vi "Interpolate.vi"(9 "offset":dbl, 10 "Target dt":dbl, 11 "input waveform":waveform(dbl)) -> (3 "output waveform":waveform(dbl))   [LabVIEW 2018, in "Waveform Equalizer.lvlib"]
uses:
  Waveform Equalizer.lvlib
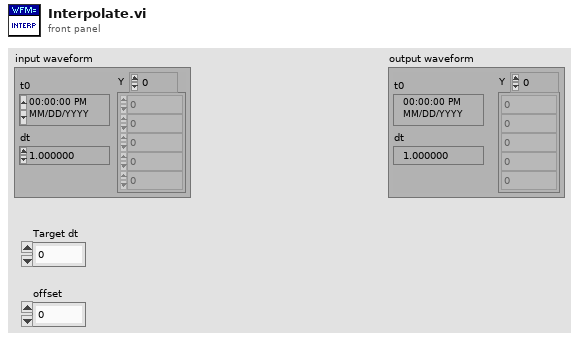
[diagram p1: front panel]
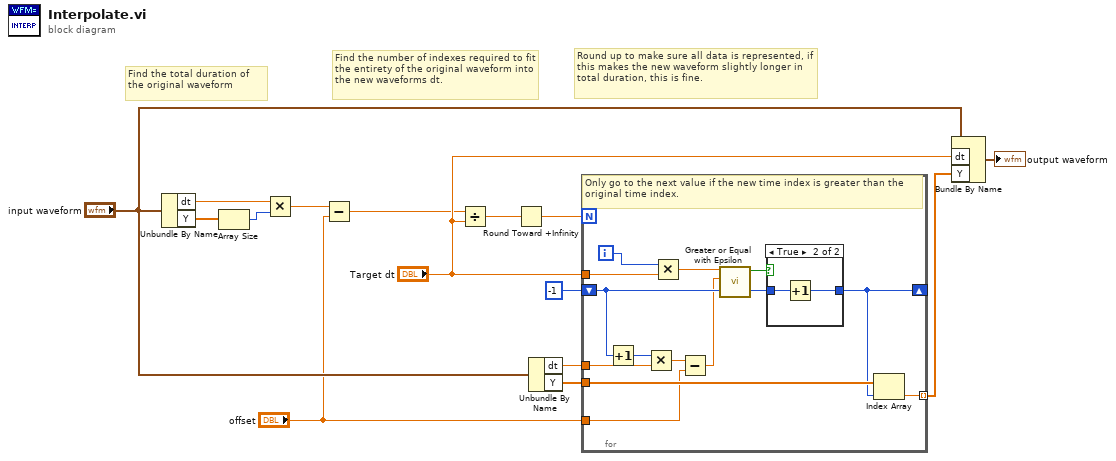
[diagram p0: block diagram]
diagram:
  # "Round up to make sure all data is represented, if this makes the new waveform slightly longer in total duration, this is fine."
  # "Find the number of indexes required to fit the entirety of the original waveform into the new waveforms dt."
  # "Find the total duration of the original waveform"
  n1 = Unbundle By Name("input waveform") -> ("dt"=w13:dbl, "Y"=w15:dbl[])
  n2 = Array Size(array=w15) -> (size(s)=w14:i32)
  n3 = Multiply(x=w13, y=w14) -> (x*y=w3:dbl)
  n4 = Subtract(x=w3, y="offset") -> (x-y=w2:dbl)
  n5 = Divide(x=w2, y="Target dt") -> (x/y=w12:dbl)
  n6 = Round Toward +Infinity(x=w12) -> (ceil(x): smallest int >= x=w11:dbl)
  n7 = Unbundle By Name("input waveform") -> ("dt"=w9:dbl, "Y"=w8:dbl[])
  n8 = for {
    N: w11 -> [_]
    tunnel: "Target dt" -> [w27]
    shift-right: [w25] -> _
    shift-left: -1 -> [w22]
    tunnel: w9 -> [w28]
    tunnel: w8 -> [w26]
    tunnel: [w24] -> w5 mode=indexing
    tunnel: "offset" -> [w16]
    i -> [w23]
    # "Only go to the next value if the new time index is greater than the original time index."
    n9 = Increment(x=w22) -> (x+1=w21:i32)
    n10 = Multiply(x=w21, y=w28) -> (x*y=w19:dbl)
    n11 = Multiply(x=w23, y=w27) -> (x*y=w20:dbl)
    n12 = Subtract(x=w19, y=w16) -> (x-y=w17:dbl)
    n13 = call "Greater or Equal with Epsilon.vi"("b"=w17, "a"=w20) -> ("a>=b"=w18:bool)  [unwired: 9 in]
    n14 = case shown="True" w18 {
      tunnel: w22 -> [w29 w31]
      tunnel: [w29 w30] -> w25
      frame False {
      }
      frame True {
        n15 = Increment(x=w31) -> (x+1=w30:i32)
      }
    }
    n16 = Index Array(array=w26, index=w25) -> (element=w24:dbl)
  }
  n17 = Bundle By Name(cluster="input waveform", "dt"="Target dt", "Y"=w5) -> (→"output waveform":waveform(dbl))
